vi "fit angle data to line.vi"(10 "length":i32=1000, 11 "remaining elements":cluster{"mean":dbl, dbl}[](array[cluster])) -> (2 "graphs":cluster{dbl[], dbl[]}[](array[cluster]), 3 "deg/hr":dbl)   [LabVIEW 2017]
uses:
  <vilib>/Analysis/baseanly.llb/Mean (DBL).vi
  <vilib>/Analysis/NI_AALBase.lvlib
  <vilib>/Analysis/NI_AALPro.lvlib
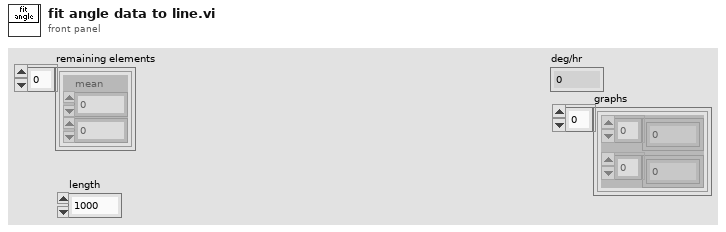
[diagram p1: front panel]
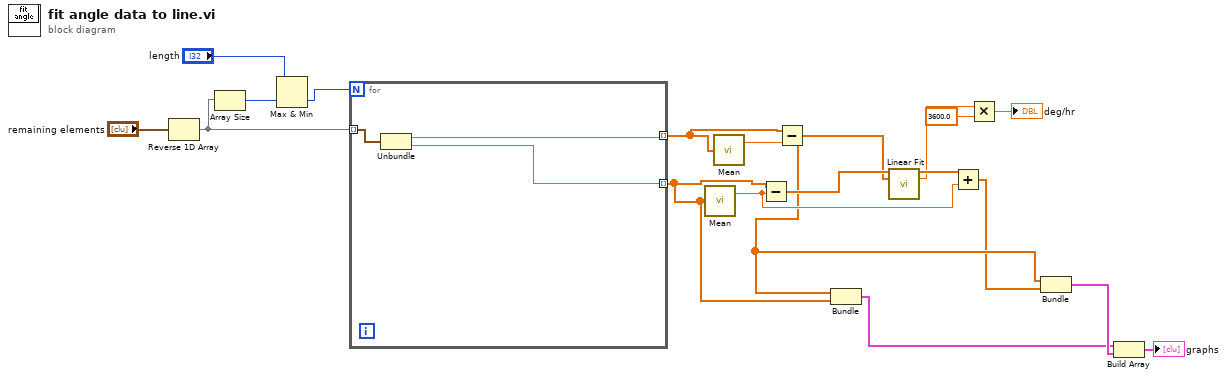
[diagram p0: block diagram]
diagram:
  n1 = Reverse 1D Array(array="remaining elements") -> (reversed array=w18:cluster{"mean":dbl, dbl}[])
  n2 = Array Size(array=w18) -> (size(s)=w17:i32)
  n3 = Max & Min(x="length", y=w17) -> (min(x,y)=w15:i32)  [unwired: 1 out]
  n4 = for {
    N: w15 -> [_]
    tunnel: w18 -> [w22] mode=indexing
    tunnel: [w21] -> w7 mode=indexing
    tunnel: [w20] -> w6 mode=indexing
    n5 = Unbundle(w22) -> ("mean"=w21:dbl, w20:dbl)
  }
  n6 = call-poly <vilib>:"Mean.vi"("X"=w6) -> ("mean"=w11:dbl)  [unwired: 1 out]
  n7 = call-poly <vilib>:"Mean.vi"("X"=w7) -> ("mean"=w14:dbl)  [unwired: 1 out]
  n8 = Subtract(x=w6, y=w11) -> (x-y=w13:dbl[])
  n9 = Subtract(x=w7, y=w14) -> (x-y=w5:dbl[])
  n10 = Bundle(w5, w6) -> (w2:cluster{dbl[], dbl[]})  [unwired: 1 in]
  n11 = call <vilib>:"Linear Fit.vi"("Y"=w13, "X"=w5) -> ("Best Linear Fit"=w12:dbl[], "slope"=w10:dbl)  [unwired: 9 in, 3 out]
  n12 = Add(x=w12, y=w11) -> (x+y=w4:dbl[])
  n13 = Multiply(x=w10, y=3600.0) -> (x*y=→"deg/hr":dbl)
  n14 = Bundle(w5, w4) -> (w3:cluster{dbl[], dbl[]})  [unwired: 1 in]
  n15 = Build Array(w2, w3) -> (→"graphs":cluster{dbl[], dbl[]}[])
